vi "coolRound.vi"(6 "Decimal Rounding (.5)":dbl=0.5, 7 "Number (0.00)":dbl) -> (3 "Rounded Number":dbl)   [LabVIEW 2011]
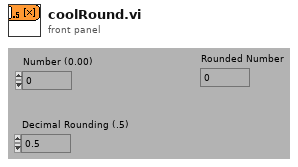
[diagram p1: front panel]
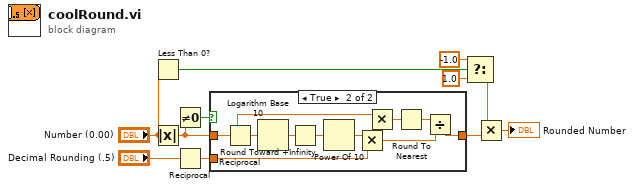
[diagram p0: block diagram]
diagram:
  n1 = Less Than 0?(x="Number (0.00)") -> (x < 0?=w6:bool)
  n2 = Absolute Value(x="Number (0.00)") -> (abs(x)=w8:dbl)
  n3 = Not Equal To 0?(x=w8) -> (x != 0?=w11:bool)
  n4 = Reciprocal(x="Decimal Rounding (.5)") -> (1/x=w10:dbl)
  n5 = case shown="True" w11 {
    tunnel: [w12 w20] -> w4
    tunnel: w8 -> [w12 w14]
    tunnel: w10 -> [_ w13]
    frame False {
    }
    frame True {
      n6 = Reciprocal(x=w14) -> (1/x=w18:dbl)
      n7 = Logarithm Base 10(1:w18) -> (0:w16:dbl)
      n8 = Round Toward +Infinity(x=w16) -> (ceil(x): smallest int >= x=w15:dbl)
      n9 = Power Of 10(x=w15) -> (10^x=w17:dbl)
      n10 = Multiply(x=w17, y=w13) -> (x*y=w19:dbl)
      n11 = Multiply(x=w14, y=w19) -> (x*y=w21:dbl)
      n12 = Round To Nearest(number=w21) -> (nearest integer value=w22:dbl)
      n13 = Divide(x=w22, y=w19) -> (x/y=w20:dbl)
    }
  }
  n14 = Select(t=-1.0, s=w6, f=1.0) -> (s? t:f=w3:dbl)
  n15 = Multiply(x=w3, y=w4) -> (x*y=→"Rounded Number":dbl)
